vi "svmdense_predict_probabilities.vi"(8 "error in (no error)":errorcluster, 10 "x":dbl[](array[numeric]), 11 "Model":T1) -> (0 "error out":errorcluster, 2 "Probability estimates":dbl[](array[numeric]), 3 "Predicted label":dbl)   [LabVIEW 2015]
doc: "This function does classification or regression on a test vector x given a model with probability information.\n\nFor a classification model with probability information, this function gives nr_class probability estimates in the output array probability estimates."
uses:
  Controls/svmdense_model.ctl
  LibSVM Sparse/Wrapper API/Controls/svm_parameter.ctl
  LibSVM Sparse/Wrapper API/Controls/svm_type.ctl
  LibSVM Sparse/Wrapper API/Controls/svm_kernel_type.ctl
  bin/x64/LabVIEW-libsvm-dense.dll
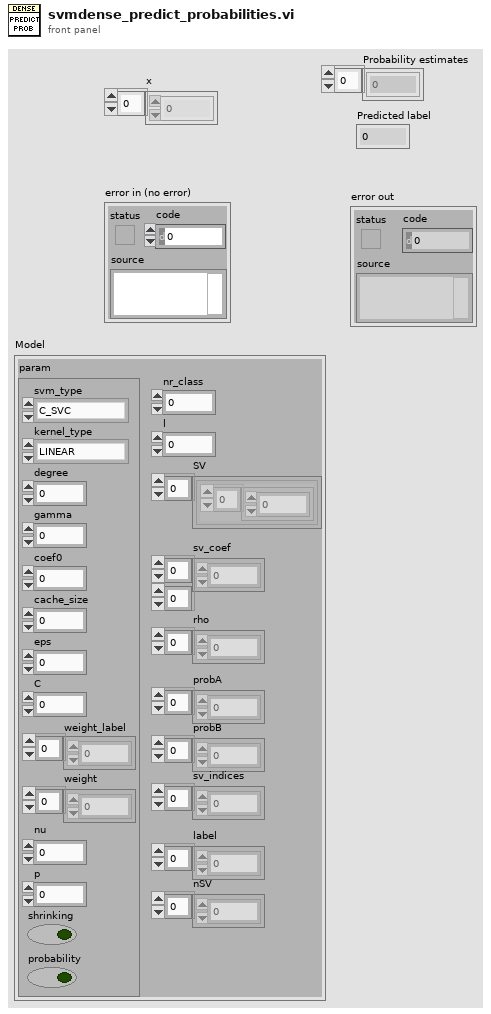
[diagram p1: front panel]
types:
  T1 = typedef "svmdense_model.ctl" = cluster{"param":T2, "nr_class":i32, "l":i32, "SV":cluster{"Array":dbl[]}[], "sv_coef":dbl[][], "rho":dbl[], "probA":dbl[], "probB":dbl[], "sv_indices":i32[], "label":i32[], "nSV":i32[]}
  T2 = typedef "svm_parameter.ctl" = cluster{"svm_type":T3, "kernel_type":T4, "degree":i32, "gamma":dbl, "coef0":dbl, "cache_size":dbl, "eps":dbl, "C":dbl, "weight_label":i32[], "weight":dbl[], "nu":dbl, "p":dbl, "shrinking":bool, "probability":bool}
  T3 = typedef "svm_type.ctl" = enum32{"C_SVC", "NU_SVC", "ONE_CLASS", "EPSILON_SVR", "NU_SVR"}
  T4 = typedef "svm_kernel_type.ctl" = enum32{"LINEAR", "POLY", "RBF", "SIGMOID", "PRECOMPUTED"}
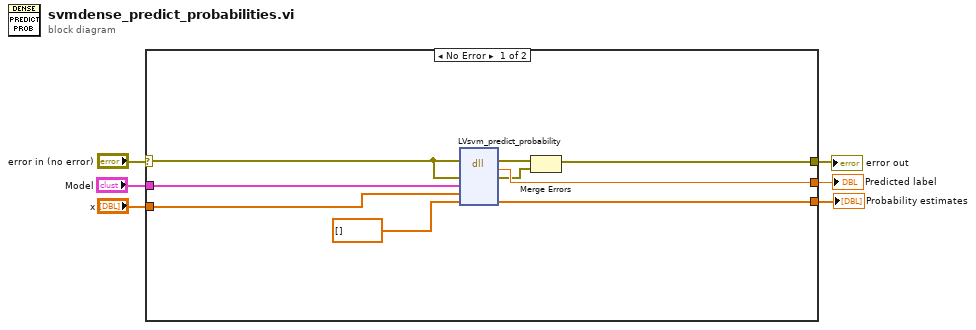
[diagram p0: block diagram]
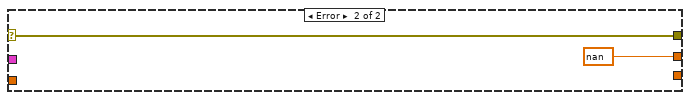
[diagram p2: hidden frame]
diagram:
  n1 = case shown="No Error" "error in (no error)" {
    selector: "error in (no error)" -> [w15 w17]
    tunnel: [w14 w17] -> w6
    tunnel: "Model" -> [w13 _]
    tunnel: "x" -> [w12 _]
    tunnel: [w11 nan ("predicted label")] -> w4
    tunnel: [w10 _] -> w3
    frame No Error {
      n2 = dll-call lib="C:/dev/LabVIEW-libsvm/LabVIEW/bin/x64/LabVIEW-libsvm-dense.dll" fn="LVsvm_predict_probability"(error in=w15, "lvErr"=w15, "model_in"=w13, "x_in"=w12, "prob_estimates_out"=dbl[] [] ("dec_values_out")) -> (error out=w9:errorcluster, "predicted label"=w11:dbl, "lvErr"=w8:errorcluster, "prob_estimates_out"=w10:dbl[])  [unwired: 4 in, 1 out]
      n3 = Merge Errors(w9, w8) -> (w14:errorcluster)
    }
    frame Error {
    }
  }
  "error out" <- w6
  "Predicted label" <- w4
  "Probability estimates" <- w3
